vi "SeCrTS-Obtain notifier display.vi"(8 "error in (no error)":errorcluster) -> (0 "error out":errorcluster, 3 "NOT DIS Out":T1)   [LabVIEW 2022 SP3]
uses:
  Control/SeCrTS-Notifier Ref.ctl
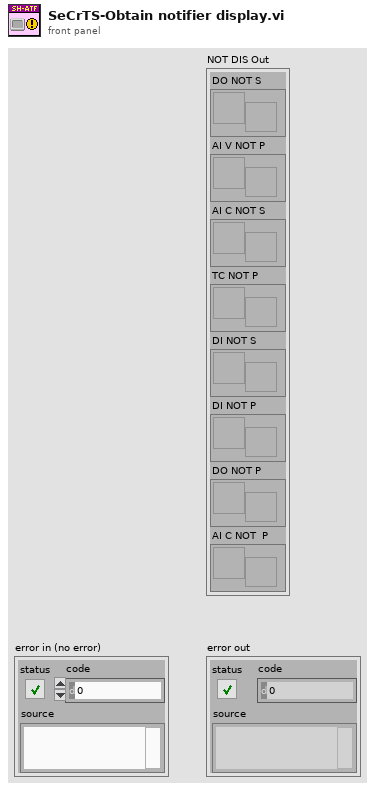
[diagram p1: front panel]
types:
  T1 = typedef "SeCrTS-Notifier Ref.ctl" = cluster{"DO NOT S":refnum<notifier>, "AI V NOT P":refnum<notifier>, "AI C NOT S":refnum<notifier>, "TC NOT P":refnum<notifier>, "DI NOT S":refnum<notifier>, "DI NOT P":refnum<notifier>, "DO NOT P":refnum<notifier>, "AI C NOT  P":refnum<notifier>}
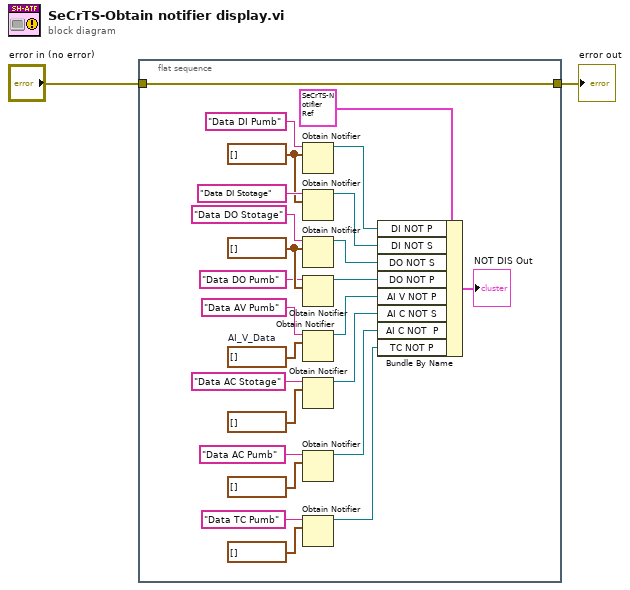
[diagram p0: block diagram]
diagram:
  n1 = flat-sequence {
    tunnel: "error in (no error)" -> [w3]
    tunnel: [w3] -> w1
    frame #0 {
      w11 = digitalwaveform[] [] ("DI_Data")
      w9 = waveform(dbl)[] [] ("AI_C_Data")
      w26 = waveform(dbl)[] []  # AI_V_Data
      n2 = Obtain Notifier(name (unnamed)="Data DI Pumb", notification data type=w11) -> (notifier out=w10:refnum<notifier>)  [unwired: 2 in, 2 out]
      n3 = Obtain Notifier(name (unnamed)="Data DI Stotage", notification data type=w11) -> (notifier out=w13:refnum<notifier>)  [unwired: 2 in, 2 out]
      n4 = Obtain Notifier(name (unnamed)="Data DO Stotage", notification data type=w9) -> (notifier out=w18:refnum<notifier>)  [unwired: 2 in, 2 out]
      n5 = Obtain Notifier(name (unnamed)="Data DO Pumb", notification data type=w9) -> (notifier out=w7:refnum<notifier>)  [unwired: 2 in, 2 out]
      n6 = Obtain Notifier(name (unnamed)="Data AV Pumb", notification data type=w26) -> (notifier out=w17:refnum<notifier>)  [unwired: 2 in, 2 out]
      n7 = Obtain Notifier(name (unnamed)="Data AC Stotage", notification data type=waveform(dbl)[] [] ("AI_C_Data")) -> (notifier out=w16:refnum<notifier>)  [unwired: 2 in, 2 out]
      n8 = Obtain Notifier(name (unnamed)="Data AC Pumb", notification data type=waveform(dbl)[] [] ("AI_C_Data")) -> (notifier out=w4:refnum<notifier>)  [unwired: 2 in, 2 out]
      n9 = Obtain Notifier(name (unnamed)="Data TC Pumb", notification data type=waveform(dbl)[] [] ("AI_C_Data")) -> (notifier out=w15:refnum<notifier>)  [unwired: 2 in, 2 out]
      n10 = Bundle By Name(cluster=T1 {"DO NOT S"=refnum, "AI V NOT P"=refnum, "AI C NOT S"=refnum, "TC NOT P"=refnum, "DI NOT S"=refnum, "DI NOT P"=refnum, "DO NOT P"=refnum, "AI C NOT  P"=refnum}, "DI NOT P"=w10, "DI NOT S"=w13, "DO NOT S"=w18, "DO NOT P"=w7, "AI V NOT P"=w17, "AI C NOT S"=w16, "AI C NOT  P"=w4, "TC NOT P"=w15) -> (→"NOT DIS Out":T1)
    }
  }
  "error out" <- w1
